vi "V7310.Main.Close.vi"(8 "error in":errorcluster, 10 "State (Init)":T1=enum."Init", 11 "Data in":T2={"Status"={"State"=enum."Init", "LaserStatus"=enum."-", "LaserStatusRaw"="", "Ref"=refnum, "RTC TS"=timestamp(0 s since 1904-01-01), "Conn TS"=timestamp(0 s since 1904-01-01), "Msg"=[], "JobInUse"="", "Jobs"=[], "Vars"=[]}, "Sets"={"Address"="192.168.2.1", "Timeout_ms"=5000, "ReconnectPeriod_s"=0, "JobInUse"="", "CoordinatesOffset"={"X"=0.0, "Y"=0.0}}}) -> (0 "error out":errorcluster, 3 "Data out":T2={"Status"={"State"=enum."Init", "LaserStatus"=enum."-", "LaserStatusRaw"="", "Ref"=refnum, "RTC TS"=timestamp(0 s since 1904-01-01), "Conn TS"=timestamp(0 s since 1904-01-01), "Msg"=[], "JobInUse"="", "Jobs"=[], "Vars"=[]}, "Sets"={"Address"="192.168.2.1", "Timeout_ms"=5000, "ReconnectPeriod_s"=0, "JobInUse"="", "CoordinatesOffset"={"X"=0.0, "Y"=0.0}}})   [LabVIEW 2016]
uses:
  V7310.Data.ctl
  V7310.Data.Status.ctl
  V7310.Data.Status.State.ctl
  LowLevel/V7310.LaserStatus.ctl
  LowLevel/V7310.Message.Data.ctl
  LowLevel/V7310.Job.Variable.ctl
  V7310.Data.Sets.ctl
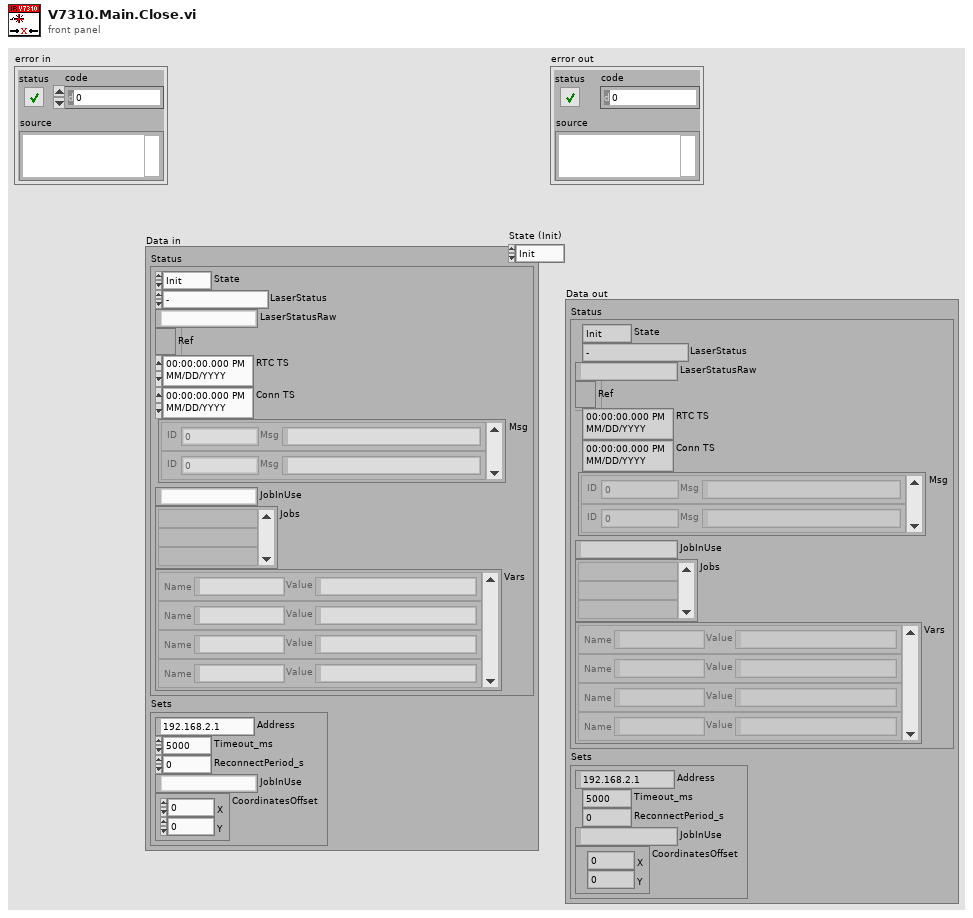
[diagram p1: front panel]
types:
  T1 = typedef "V7310.Data.Status.State.ctl" = enum16{"First", "Init", "Msg", "Error", "Abort", "Idle", "Run"}
  T2 = typedef "V7310.Data.ctl" = cluster{"Status":T3, "Sets":T7}
  T3 = typedef "V7310.Data.Status.ctl" = cluster{"State":T1, "LaserStatus":T4, "LaserStatusRaw":string, "Ref":refnum<k5>, "RTC TS":timestamp, "Conn TS":timestamp, "Msg":T5[], "JobInUse":string, "Jobs":string[], "Vars":T6[]}
  T4 = typedef "V7310.LaserStatus.ctl" = enum16{"-", "FatalError", "Initialize", "KeySwitchOpen", "TimeoutInterlock", "InterlockOpen", "StartUp", "ShutterlockOpen", "Standby", "Ready", "PrepareForMarking", "WaitForTrigger", "Marking"}
  T5 = typedef "V7310.Message.Data.ctl" = cluster{"ID":i32, "Msg":string}
  T6 = typedef "V7310.Job.Variable.ctl" = cluster{"Name":string, "Value":string}
  T7 = typedef "V7310.Data.Sets.ctl" = cluster{"Address":string, "Timeout_ms":i32, "ReconnectPeriod_s":i32, "JobInUse":string, "CoordinatesOffset":cluster{"X":dbl, "Y":dbl}}
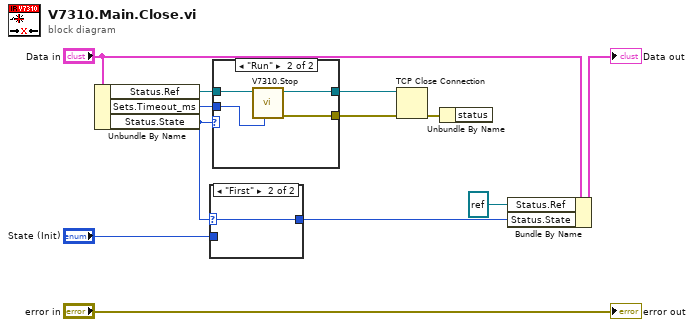
[diagram p0: block diagram]
diagram:
  n1 = Unbundle By Name("Data in") -> ("Status.Ref"=w8:refnum<k5>, "Sets.Timeout_ms"=w4:i32, "Status.State"=w1:T1)
  n2 = case shown="\"First\"" w1 {
    selector: w1 -> [_ w14]
    tunnel: [w13 w14] -> w3
    tunnel: "State (Init)" -> [w13 _]
    frame Default {
    }
    frame "First" {
    }
  }
  n3 = case shown="\"Run\"" w1 {
    tunnel: w8 -> [w15 w19]
    tunnel: [w15 w18] -> w7
    tunnel: [_ w17] -> w6
    tunnel: w4 -> [_ w16]
    frame Default {
    }
    frame "Run" {
      n4 = call "V7310.Stop.vi"("timeout ms (5000)"=w16, "Connection in"=w19) -> ("error out"=w17:errorcluster, "Connection out"=w18:refnum<k5>)  [unwired: 8 in]
    }
  }
  n5 = TCP Close Connection(connection ID=w7, error in (no error)=w6) -> (error out=w5:errorcluster)  [unwired: 1 in, 1 out]
  n6 = Unbundle By Name(w5) -> ()  [unwired: 1 out]
  n7 = Bundle By Name(cluster="Data in", "Status.Ref"=refnum<k5> refnum, "Status.State"=w3) -> (→"Data out":T2)
  "error out" <- "error in"
